vi "Read Is Server.vi"(8 "error in (no error)":errorcluster, 11 "WebSocket Client in":refnum<class "WebSocket Client.lvclass">) -> (0 "error out":errorcluster, 2 "Is Server?":bool, 3 "WebSocket Client out":refnum<class "WebSocket Client.lvclass">)   [LabVIEW 2013, in "WebSockets.lvlib" / "WebSocket Client.lvclass"]
uses:
  WebSocket Client.lvclass
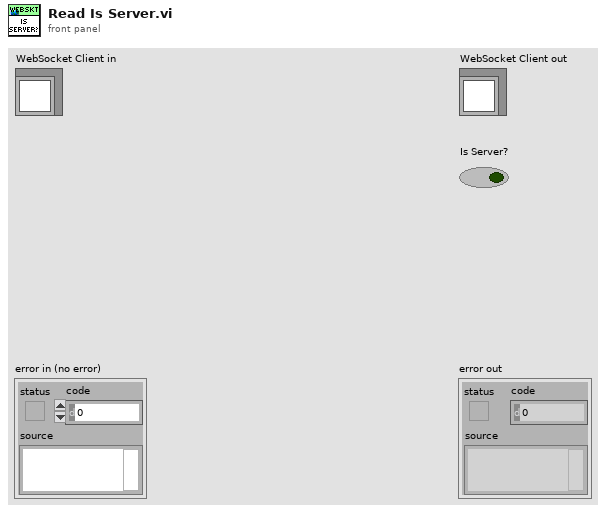
[diagram p1: front panel]
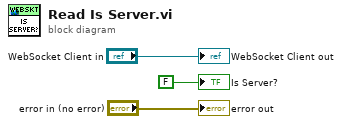
[diagram p0: block diagram]
diagram:
  "error out" <- "error in (no error)"
  "WebSocket Client out" <- "WebSocket Client in"
  "Is Server?" <- FALSE ("Is Server?")
